vi "BrakeAndDriveSet.vi"(5 "Drive Torque":dbl format="%#_13g", 7 "Drive Velocity":dbl format="%#_13g", 8 "error in (no error)":errorcluster, 9 "Brake Torque":dbl format="%#_13g", 10 "Brake Velocity":dbl format="%#_13g", 11 "Queue in":refnum<queue>) -> (0 "error out":errorcluster, 3 "Queue out":refnum<queue>)   [LabVIEW 2026, in "Acquisition.lvlib"]
uses:
  Acquisition/Acquisition.lvlib
  support/Message Queue/Message Cluster.ctl
  support/Message Queue/Message Queue.lvlib
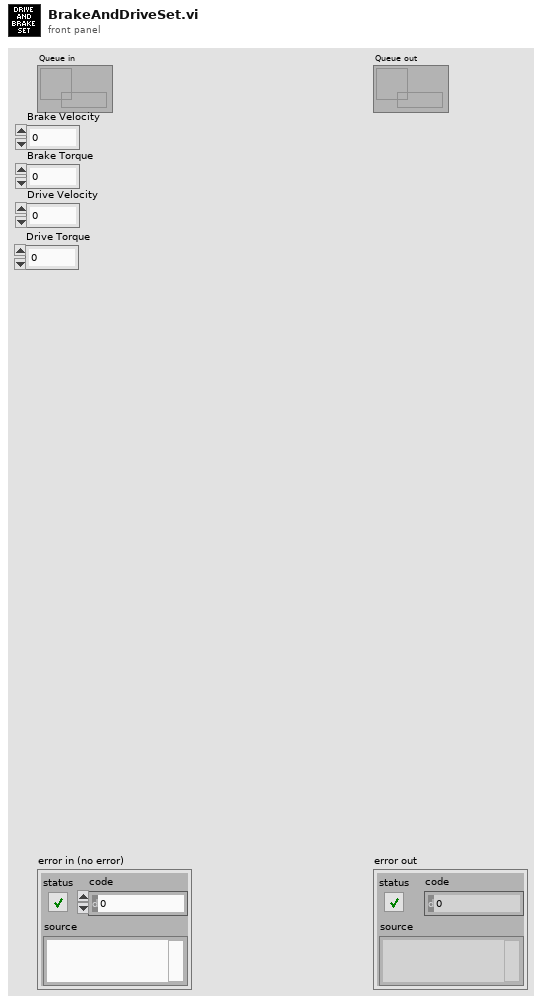
[diagram p1: front panel]
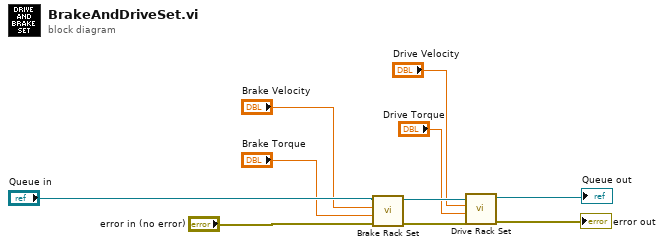
[diagram p0: block diagram]
diagram:
  n1 = call "Brake Rack Set.vi"("error in"="error in (no error)", "Torque"="Brake Torque", "Velocity"="Brake Velocity", "queue"="Queue in") -> ("error out"=w1:errorcluster, "dup Message Queue"=w9:refnum<queue>)  [unwired: 6 in]
  n2 = call "Drive Rack Set.vi"("error in"=w1, "Torque"="Drive Torque", "Velocity"="Drive Velocity", "queue"=w9) -> ("error out"=→"error out":errorcluster, "dup Message Queue"=→"Queue out":refnum<queue>)  [unwired: 6 in]
